vi "SPC_read_parameters_from_inifile.vi"(6 "Ini file path & name":string="C:\\Program Files (x86)\\BH\\SPCM\\DLL\\spcm.ini", 8 "Error In":errorcluster, 11 "DLL Path":path) -> (0 "Error Out":errorcluster, 3 "DLL Path":path, 4 "SPCdata":T1={"base_adr"=896, "init"=0, "cfd_limit_low"=0.0, "cfd_limit_high"=5.0, "cfd_zc_level"=80.0, "cfd_holdoff"=0.0, "sync_zc_level"=5.0, "sync_holdoff"=0.0, "sync_threshold"=1.0, "tac_range"=4.0, "sync_freq_div"=-20, "tac_gain"=50, "tac_offset"=1.0, "tac_limit_low"=0.0, "tac_limit_high"=10.0, "adc_resolution"=80, "ext_latch_delay"=10, "collect_time"=0.0, "display_time"=0.01, "repeat_time"=1.0, "stop_on_time"=10, "stop_on_ovfl"=1, "dither_range"=1, "count_incr"=0, "mem_bank"=1, "dead_time_comp"=0, "scan_control"=1, "routing_mode"=61440, "tac_enable_hold"=0.0, "pci_card_no"=10, "mode"=65535, "scan_size_x"=0, "scan_size_y"=1, "scan_rout_x"=1, "scan_rout_y"=1, "scan_flyback"=1, "scan_borders"=0, "scan_polarity"=0, "pixel_clock"=0, "line_compression"=0, "trigger"=0, "pixel_time"=1.0, "ext_pixclk_div"=0, "rate_count_time"=1.0, "macro_time_clk"=1, "add_select"=0, "test_eep"=0, "adc_zoom"=0, "img_size_x"=1, "img_size_y"=1, "img_rout_x"=1, "img_rout_y"=1, "xy_gain"=1, "master_clock"=0, "adc_sample_delay"=0, "detector_type"=1, "chan_enable"=0, "chan_slope"=0, "chan_spec_no"=0, "tdc_control"=4294936595, "tdc_offset1"=0.0, "tdc_offset2"=0.0, "tdc_offset3"=0.0, "tdc_offset4"=0.0, "future_reserve1"=0, "future_reserve2"=0, "future_reserve3"=0, "future_reserve4"=0, "future_reserve5"=0, "future_reserve6"=0, "future_reserve7"=0})   [LabVIEW 2019]
doc: "The procedure reads parameters from the file ‘inifile’ and transfers them to the ‘SPCdata’ structure ‘data’.\nThe ‘inifile’ file is an ASCII file with a structure shown in SPC_init description. We recommend to use either the original .ini files or the files created using function SPC_save_parameters_to_inifile. \nIf a particular parameter is not present in .ini file or cannot be read, the appropriate field in SPCdata ‘data’ structure is set to the parameter’s default value.\nUse SPC_set_parameters to send result parameters set to the SPC module.\n\ninfo@becker-hickl.com"
uses:
  SPC_Controls/SPCdata.ctl
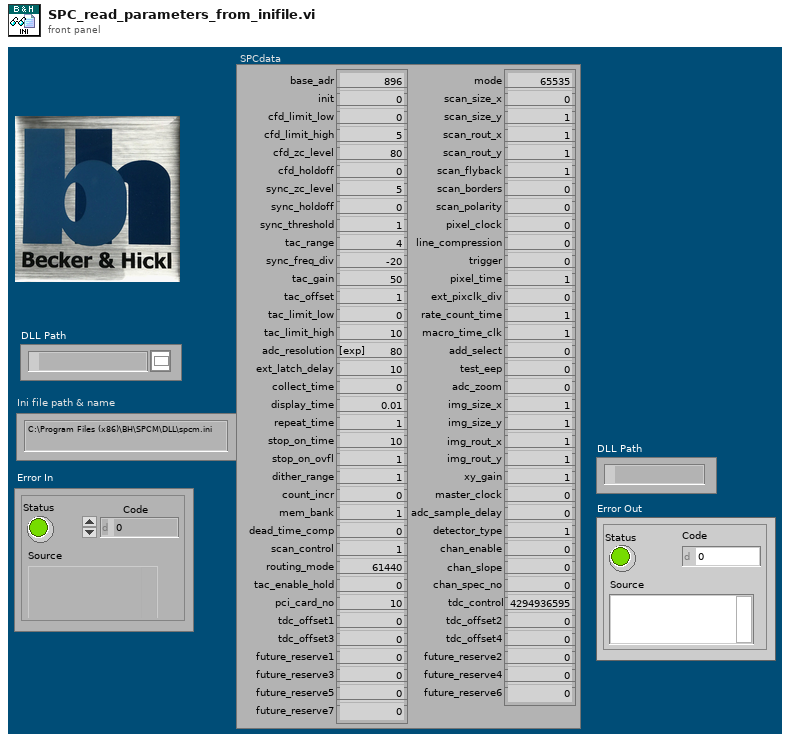
[diagram p1: front panel]
types:
  T1 = typedef "SPCdata.ctl" = cluster{"base_adr":u16, "init":i16, "cfd_limit_low":sgl, "cfd_limit_high":sgl, "cfd_zc_level":sgl, "cfd_holdoff":sgl, "sync_zc_level":sgl, "sync_holdoff":sgl, "sync_threshold":sgl, "tac_range":sgl, "sync_freq_div":i16, "tac_gain":i16, "tac_offset":sgl, "tac_limit_low":sgl, "tac_limit_high":sgl, "adc_resolution":i16, "ext_latch_delay":i16, "collect_time":sgl, "display_time":sgl, "repeat_time":sgl, "stop_on_time":i16, "stop_on_ovfl":i16, "dither_range":i16, "count_incr":i16, "mem_bank":i16, "dead_time_comp":i16, "scan_control":u16, "routing_mode":u16, "tac_enable_hold":sgl, "pci_card_no":i16, "mode":u16, "scan_size_x":u32, "scan_size_y":u32, "scan_rout_x":u32, "scan_rout_y":u32, "scan_flyback":u32, "scan_borders":u32, "scan_polarity":u16, "pixel_clock":u16, "line_compression":u16, "trigger":u16, "pixel_time":sgl, "ext_pixclk_div":u32, "rate_count_time":sgl, "macro_time_clk":i16, "add_select":i16, "test_eep":i16, "adc_zoom":i16, "img_size_x":u32, "img_size_y":u32, "img_rout_x":u32, "img_rout_y":u32, "xy_gain":i16, "master_clock":i16, "adc_sample_delay":i16, "detector_type":i16, "chan_enable":u32, "chan_slope":u32, "chan_spec_no":u32, "tdc_control":u32, "tdc_offset1":sgl, "tdc_offset2":sgl, "tdc_offset3":sgl, "tdc_offset4":sgl, "future_reserve1":u64, "future_reserve2":u64, "future_reserve3":u64, "future_reserve4":u64, "future_reserve5":u64, "future_reserve6":u64, "future_reserve7":u64}
  T2 = typedef "SPCdata.ctl" = cluster{"base_adr":u16, "init":i16, "cfd_limit_low":sgl, "cfd_limit_high":sgl, "cfd_zc_level":sgl, "cfd_holdoff":sgl, "sync_zc_level":sgl, "sync_holdoff":sgl, "sync_threshold":sgl, "tac_range":sgl, "sync_freq_div":i16, "tac_gain":i16, "tac_offset":sgl, "tac_limit_low":sgl, "tac_limit_high":sgl, "adc_resolution":i16, "ext_latch_delay":i16, "collect_time":sgl, "display_time":sgl, "repeat_time":sgl, "stop_on_time":i16, "stop_on_ovfl":i16, "dither_range":i16, "count_incr":i16, "mem_bank":i16, "dead_time_comp":i16, "scan_control":u16, "routing_mode":u16, "tac_enable_hold":sgl, "pci_card_no":i16, "mode":u16, "scan_size_x":u32, "scan_size_y":u32, "scan_rout_x":u32, "scan_rout_y":u32, "scan_flyback":u32, "scan_borders":u32, "scan_polarity":u16, "pixel_clock":u16, "line_compression":u16, "trigger":u16, "pixel_time":sgl, "ext_pixclk_div":u32, "rate_count_time":sgl, "macro_time_clk":i16, "add_select":i16, "test_eep":i16, "adc_zoom":i16, "img_size_x":u32, "img_size_y":u32, "img_rout_x":u32, "img_rout_y":u32, "xy_gain":i16, "master_clock":i16, "adc_sample_delay":i16, "detector_type":i16, "chan_enable":u32, "chan_slope":u32, "chan_spec_no":u32, "x_axis_type":i16, "tdc_offset1":sgl, "tdc_offset2":sgl, "tdc_offset3":sgl, "tdc_offset4":sgl}
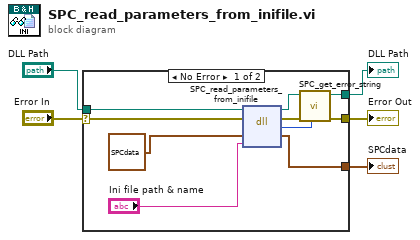
[diagram p0: block diagram]
diagram:
  n1 = case shown="No Error" "Error In" {
    selector: "Error In" -> [w12 w17]
    tunnel: [w9 w16] -> w5
    tunnel: [w14 w17] -> w4
    tunnel: "DLL Path" -> [w11 w16]
    tunnel: [w7 _] -> w1
    frame No Error {
      n2 = dll-call lib="D:/spcm/lib/lab_view/lv10.0/spcm32.dll" fn="SPC_read_parameters_from_inifile"(path in=w11, error in=w12, T2 {"base_adr"=896, "init"=0, "cfd_limit_low"=0.0, "cfd_limit_high"=5.0, "cfd_zc_level"=80.0, "cfd_holdoff"=0.0, "sync_zc_level"=5.0, "sync_holdoff"=0.0, "sync_threshold"=1.0, "tac_range"=4.0, "sync_freq_div"=-20, "tac_gain"=50, "tac_offset"=1.0, "tac_limit_low"=0.0, "tac_limit_high"=10.0, "adc_resolution"=80, "ext_latch_delay"=10, "collect_time"=0.0, "display_time"=0.01, "repeat_time"=1.0, "stop_on_time"=10, "stop_on_ovfl"=1, "dither_range"=1, "count_incr"=0, "mem_bank"=1, "dead_time_comp"=0, "scan_control"=1, "routing_mode"=61440, "tac_enable_hold"=0.0, "pci_card_no"=10, "mode"=65535, "scan_size_x"=0, "scan_size_y"=1, "scan_rout_x"=1, "scan_rout_y"=1, "scan_flyback"=1, "scan_borders"=0, "scan_polarity"=0, "pixel_clock"=0, "line_compression"=0, "trigger"=0, "pixel_time"=1.0, "ext_pixclk_div"=0, "rate_count_time"=1.0, "macro_time_clk"=1, "add_select"=0, "test_eep"=0, "adc_zoom"=0, "img_size_x"=1, "img_size_y"=1, "img_rout_x"=1, "img_rout_y"=1, "xy_gain"=1, "master_clock"=0, "adc_sample_delay"=0, "detector_type"=1, "chan_enable"=0, "chan_slope"=0, "chan_spec_no"=0, "x_axis_type"=-30701, "tdc_offset1"=0.0, "tdc_offset2"=0.0, "tdc_offset3"=0.0, "tdc_offset4"=0.0} ("SPCdata"), "ini_file"="Ini file path & name") -> (path out=w10:path, error out=w13:errorcluster, "return type"=w8:i16, w7:T2)  [unwired: 2 in]
      n3 = call "SPC_get_error_string.vi"("ErrorID"=w8, "Error In"=w13, "DLL Path"=w10) -> ("Error Out"=w14:errorcluster, "DLL Path"=w9:path)  [unwired: 6 in, 1 out]
    }
    frame Error {
    }
  }
  "DLL Path" <- w5
  "Error Out" <- w4
  "SPCdata" <- w1
